vi "read.vi"(7 "timeout (ms)":i32, 8 "error in (no error)":errorcluster, 9 "number of channels":i32, 10 "block size":i32, 11 "GenericFPGAWrapper in":refnum<class "GenericFPGAWrapper.lvclass">) -> (0 "error out":errorcluster, 1 "channels raw data block":T1, 2 "FIFO full?":bool, 3 "GenericFPGAWrapper out":refnum<class "GenericFPGAWrapper.lvclass">, 4 "timed out?":bool)   [LabVIEW 2010, in "GenericFPGAWrapper.lvclass"]
uses:
  GenericFPGAWrapper.lvclass
  common/arrays/pixel_raw_data_array.ctl
panel:
  out "Elements Remaining FIFO2":u32
  out "Elements Remaining FIFO1":u32
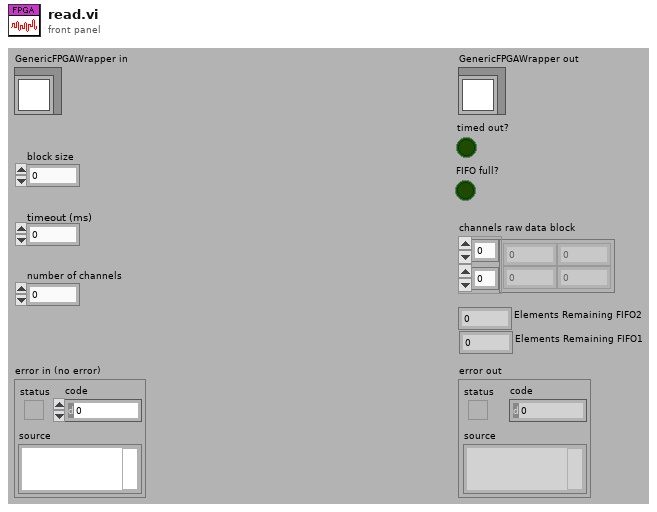
[diagram p1: front panel]
types:
  T1 = typedef "pixel_raw_data_array.ctl" = dbl[][]
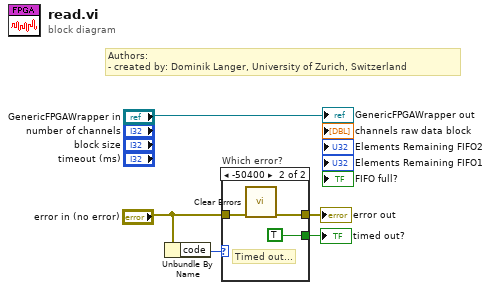
[diagram p0: block diagram]
diagram:
  # "Authors: \n- created by: Dominik Langer, University of Zurich, Switzerland"
  n1 = Unbundle By Name("error in (no error)") -> ("code"=w5:i32)
  n2 = case "Which error?" shown="-50400" w5 {
    tunnel: [w6 w8] -> w3
    tunnel: "error in (no error)" -> [w6 w9]
    tunnel: [_ TRUE] -> w1
    frame 0, Default {
    }
    frame -50400 {
      # "Timed out..."
      n3 = call <vilib>:"Clear Errors.vi"("error in (no error)"=w9) -> ("error out"=w8:errorcluster)  [unwired: 6 in]
    }
  }
  "error out" <- w3
  "timed out?" <- w1
  "GenericFPGAWrapper out" <- "GenericFPGAWrapper in"
